vi "Vision Research Phantom Series PhInt PhIHtoBITMAPINFOHEADER.vi"(0 "IH":T2, 5 "Error In (no error)":errorcluster) -> (14 "BITMAPINFOHEADER":T1, 19 "Error Out":errorcluster)   [LabVIEW 2013, in "VRI.lvlib"]
doc: "PhIHtoBITMAPINFOHEADER\nHRESULT PhIHtoBITMAPINFOHEADER(PIH pIH, PBITMAPINFOHEADER pBMIH); \n\nParameters \npIH \n Source header of the processed image.\npBMIH \n Destination header of the processed image.\nReturn \n void"
uses:
  VRI.lvlib
  _Type Defs/BITMAPINFOHEADER.ctl
  Phantom DLLs/PhInt.dll
panel:
  # "For instructions on the use of this VI, press Ctrl+H to display the help window and move the mouse over the icon, controls, and indicators"
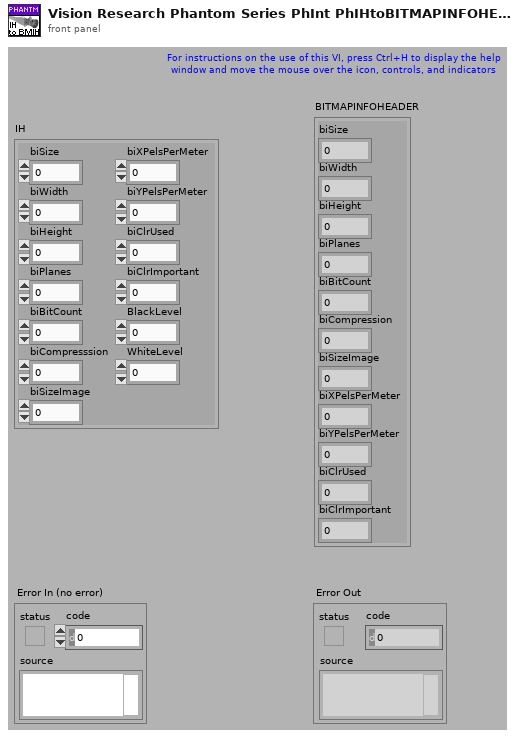
[diagram p1: front panel]
types:
  T1 = typedef "VRI.lvlib/BITMAPINFOHEADER.ctl" = cluster{"biSize":u32, "biWidth":i32, "biHeight":i32, "biPlanes":u16, "biBitCount":u16, "biCompression":u32, "biSizeImage":u32, "biXPelsPerMeter":i32, "biYPelsPerMeter":i32, "biClrUsed":u32, "biClrImportant":u32}
  T2 = cluster{"biSize":u32, "biWidth":i32, "biHeight":i32, "biPlanes":u16, "biBitCount":u16, "biCompresssion":u32, "biSizeImage":u32, "biXPelsPerMeter":i32, "biYPelsPerMeter":i32, "biClrUsed":u32, "biClrImportant":u32, "BlackLevel":i32, "WhiteLevel":i32}
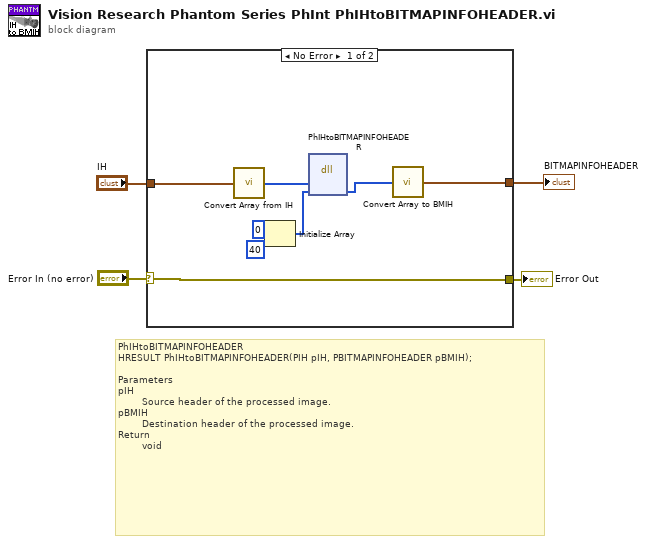
[diagram p0: block diagram]
diagram:
  # "PhIHtoBITMAPINFOHEADER\nHRESULT PhIHtoBITMAPINFOHEADER(PIH pIH, PBITMAPINFOHEADER pBMIH); \n\nParameters     \npIH                   \n        Source header of the processed image.\npBMIH             \n        Destination header of the processed image.\nReturn             \n        void"
  n1 = case shown="No Error" "Error In (no error)" {
    selector: "Error In (no error)" -> [w12 w13]
    tunnel: [w12 w13] -> w3
    tunnel: "IH" -> [w11 _]
    tunnel: [w10 _] -> w1
    frame No Error {
      n2 = call "Convert Array from IH.vi"("IH"=w11) -> ("Array"=w9:u8[])
      n3 = Initialize Array(u8 0 ("element"), 40 ("dimension size")) -> (w5:u8[])
      n4 = dll-call lib="C:/Projects/SDK/32-bit/Vision Research Phantom Series Labview Driver/Phantom DLLs/PhInt.dll" fn="PhIHtoBITMAPINFOHEADER"("pIH"=w9, "pBMIH"=w5) -> ("pBMIH"=w8:u8[])  [unwired: 4 in, 3 out]
      n5 = call "Convert Array to BMIH.vi"("Array"=w8) -> ("BITMAPINFOHEADER"=w10:T1)
    }
    frame Error {
    }
  }
  "Error Out" <- w3
  "BITMAPINFOHEADER" <- w1
